vi "Framework PPL Test.vi"() -> ()   [LabVIEW 2017]
uses:
  Built/DSF.Engine.lvlibp/Shared/Typedefs/DSF.Shared.Typedefs.Data Type.ctl
  Built/DSF.Engine.lvlibp/Shared/Typedefs/DSF.Shared.Typedefs.Direction.ctl
  Built/DSF.Engine.lvlibp/Shared/Typedefs/DSF.Shared.Typedefs.Cycle Timing Factors.ctl
  Built/DSF.Engine.lvlibp/Engine/Classes/Framework/DSF.Engine.Framework.lvclass
  <vilib>/Platform/TimedLoop/XDataNode/timing_clust.ctl
  <vilib>/Platform/TimedLoop/XDataNode/nitl_modes.ctl
  <vilib>/Platform/TimedLoop/XDataNode/wakeup.ctl
  Built/DSF.Engine.lvlibp/Engine/Classes/Debug/DSF.Engine.Debug Flags.FIFO.lvclass
  Built/DSF.Engine.lvlibp/Engine/Classes/Debug/DSF.Engine.Debug Flags.lvclass
  Built/Memory Manager.lvlibp/1abvi3w/vi.lib/National Instruments/Memory Manager/Classes/Pointer/Memory.Pointer.New.4B.vi
  Built/Memory Manager.lvlibp/1abvi3w/vi.lib/National Instruments/Memory Manager/Classes/Pointer/Memory.Pointer.Write.0D.U32.vi
  Built/Memory Manager.lvlibp/1abvi3w/vi.lib/National Instruments/Memory Manager/Classes/Pointer/Memory.Pointer.New.1B.vi
  Built/Memory Manager.lvlibp/1abvi3w/vi.lib/National Instruments/Memory Manager/Classes/Pointer/Memory.Pointer.Write.0D.Bool.vi
  Built/Memory Manager.lvlibp/1abvi3w/vi.lib/National Instruments/Memory Manager/Classes/Pointer/Memory.Pointer.Read.0D.Bool.vi
  Built/Memory Manager.lvlibp/1abvi3w/vi.lib/National Instruments/Memory Manager/Classes/Pointer/Memory.Pointer.Read.0D.I32.vi
  Built/Memory Manager.lvlibp/1abvi3w/vi.lib/National Instruments/Memory Manager/Classes/Pointer/Memory.Pointer.Read.0D.U32.vi
  Built/Memory Manager.lvlibp/1abvi3w/vi.lib/National Instruments/Memory Manager/Classes/Pointer/Memory.Pointer.Write.0D.I32.vi
  <vilib>/platform/TimedLoop/XDataNode/XDataNode.xnode
  <vilib>/Platform/TimedLoop/XDataNode/XDNodeRunTimeDep.lvlib
  Built/Memory Manager.lvlibp/1abvi3w/vi.lib/National Instruments/Memory Manager/Classes/Pointer/Memory.Pointer.lvclass
  Built/DSF.Engine.lvlibp/Shared/Classes/Framework/DSF.Shared.Configuration.Framework.lvclass
  Built/DSF.Engine.lvlibp/Engine/Classes/Pointer/DSF.Engine.Pointer.DBL.lvclass
  Built/DSF.Engine.lvlibp/Engine/Classes/Status/DSF.Engine.Status.Framework.lvclass
  Built/DSF.Engine.lvlibp/Engine/Classes/Status/DSF.Engine.Status.Framework.Performance.lvclass
  Built/DSF.Engine.lvlibp
panel:
  out "UDP Rx Port 4":u16
  out "UDP Rx Bytes 4":i32
  out "UDP Rx Count 4":i32
  out "UDP Rx Port 3":u16
  out "UDP Rx Bytes 3":i32
  out "UDP Rx Count 3":i32
  in  "infinite timeouts":bool
  out "Framework Error":errorcluster
  out "Tx duration":u32 format="%d us"
  out "Rx duration":u32 format="%d us"
  out "Actual PCL Frequency":dbl format="%.0pHz"
  out "UDP Rx Count 2":i32
  out "UDP Rx Count 1":i32
  out "UDP Rx Port 2":u16
  out "UDP Rx Bytes 2":i32
  out "UDP Rx Bytes 1":i32
  out "UDP Rx Port 1":u16
  in  "Transceiver Count":i32=4
  in  "Plugins":T4(array[cluster])=[{"plugin class"="udp", "channel count per transfer"=100, "transfer configs per group"=[{"random types?"=FALSE, "non-random type"=enum."DBL"}], "group configs"=[{"direction"=enum."Tx", "timing"={"Priority"=100, "Decimation"=1, "Offset"=0}}, {"direction"=enum."Tx", "timing"={"Priority"=100, "Decimation"=2, "Offset"=0}}, {"direction"=enum."Tx", "timing"={"Priority"=100, "Decimation"=3, "Offset"=0}}, {"direction"=enum."Tx", "timing"={"Priority"=100, "Decimation"=4, "Offset"=0}}], "plugin timing"={"Priority"=100, "Decimation"=1, "Offset"=0}}]
  in  "Configuration Path":path=path "C:/Users/Admin/Desktop/test.json"
  out "Framework Iteration":i32 format="%d cycles"
  out "Actual Period":u32 format="%d us"
  in  "Target PCL Frequency":dbl=100.0 caption="Target Period" format="%.0pHz"
  in  "stop":bool
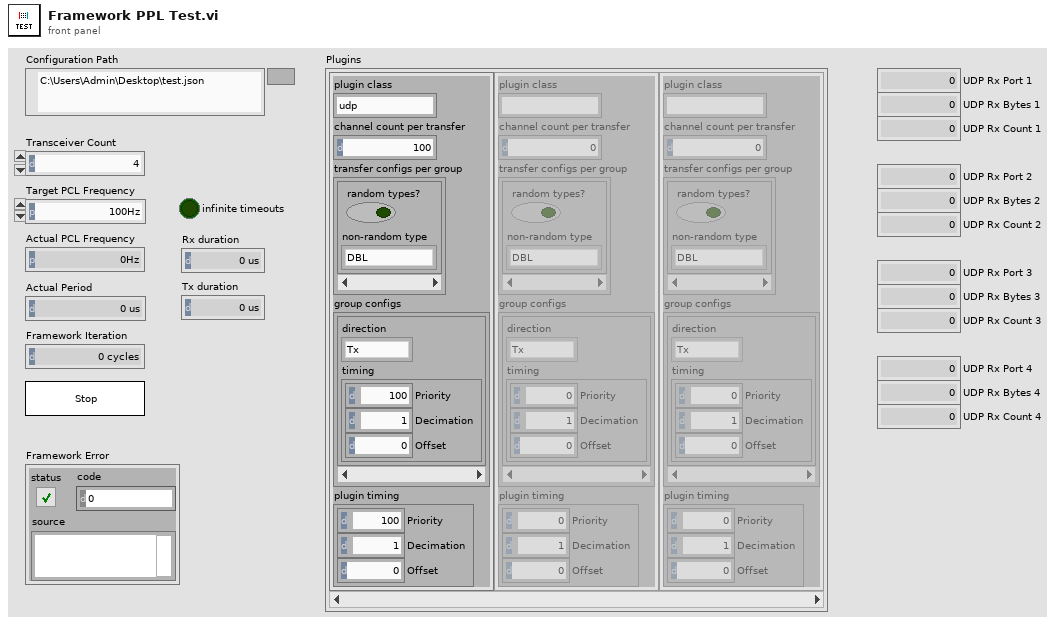
[diagram p1: front panel]
types:
  T1 = typedef "DSF.Engine.lvlibp/DSF.Shared.Typedefs.Data Type.ctl" = enum8{"Bool", "SGL", "DBL", "I8", "I16", "I32", "I64", "U8", "U16", "U32", "U64"}
  T2 = typedef "DSF.Engine.lvlibp/DSF.Shared.Typedefs.Direction.ctl" = enum8{"Tx", "Rx"}
  T3 = typedef "DSF.Engine.lvlibp/DSF.Shared.Typedefs.Cycle Timing Factors.ctl" = cluster{"Priority":u64, "Decimation":u64, "Offset":u64}
  T4 = cluster{"plugin class":string, "channel count per transfer":i32, "transfer configs per group":cluster{"random types?":bool, "non-random type":T1}[], "group configs":cluster{"direction":T2, "timing":T3}[], "plugin timing":T3}[]
  T5 = typedef "DSF.Engine.lvlibp/DSF.Shared.Refactor.Typedefs.Framework Configuration.Aggregate.ctl" = cluster{"Plugins":T6[]}
  T6 = typedef "DSF.Engine.lvlibp/DSF.Shared.Refactor.Typedefs.Plugin Configuration.Aggregate.ctl" = cluster{"name":string, "class":string, "cycle timing":T3, "Transfer Groups":T7[]}
  T7 = typedef "DSF.Engine.lvlibp/DSF.Shared.Refactor.Typedefs.Transfer Group Configuration.Aggregate.ctl" = cluster{"name":string, "direction":T2, "cycle timing":T3, "Transfers":T8[]}
  T8 = typedef "DSF.Engine.lvlibp/DSF.Shared.Refactor.Typedefs.Transfer Configuration.ctl" = cluster{"name":string, "byte order":T9, "channel configurations":T10[]}
  T9 = typedef "DSF.Engine.lvlibp/DSF.Shared.Typedefs.Byte Order.ctl" = enum8{"big-endian", "little-endian"}
  T10 = typedef "DSF.Engine.lvlibp/DSF.Shared.Refactor.Typedefs.Channel Array Configuration.ctl" = cluster{"name":string, "data type":T1, "count":u64, "buffer offset":u64, "engine offset":u64}
  T11 = typedef "XDNodeRunTimeDep.lvlib/timing_clust.ctl" = cluster{"Expected End [f-1]":u64, "Actual End [f-1]":u64, "Finished Late? [f-1]":bool, "Expected End [i-1]":u64, "Actual End [i-1]":u64, "Finished Late? [i-1]":bool, "Expected Start [i]":u64, "Actual Start [i]":u64, "Expected Start [f]":u64, "Actual Start [f]":u64, "Source Name":string, "Structure Name":string, "Period":i64, "Deadline":i64, "Offset":i64, "Start":i64, "Priority":i32, "Timeout":i32, "Mode":T12, "Wakeup Reason":T13, "Error":errorcluster, "Source Type":string, "Secondary Source Type":string, "Global End Time":u64, "Global Start Time":u64, "Frame Duration":u64, "Iteration Duration":u64, "Assigned CPU":i32, "I/O Scan Engine Mode":u32}
  T12 = typedef "XDNodeRunTimeDep.lvlib/nitl_modes.ctl" = enum32{"No Change", "Process missed periods, maintain original phase", "Discard missed periods, maintain original phase", "Process missed periods, ignore original phase", "Discard missed periods, ignore original phase"}
  T13 = typedef "XDNodeRunTimeDep.lvlib/wakeup.ctl" = enum32{"Normal", "Aborted", "Asynchronous wakeup", "Timing source error", "Timed loop error", "Timeout"}
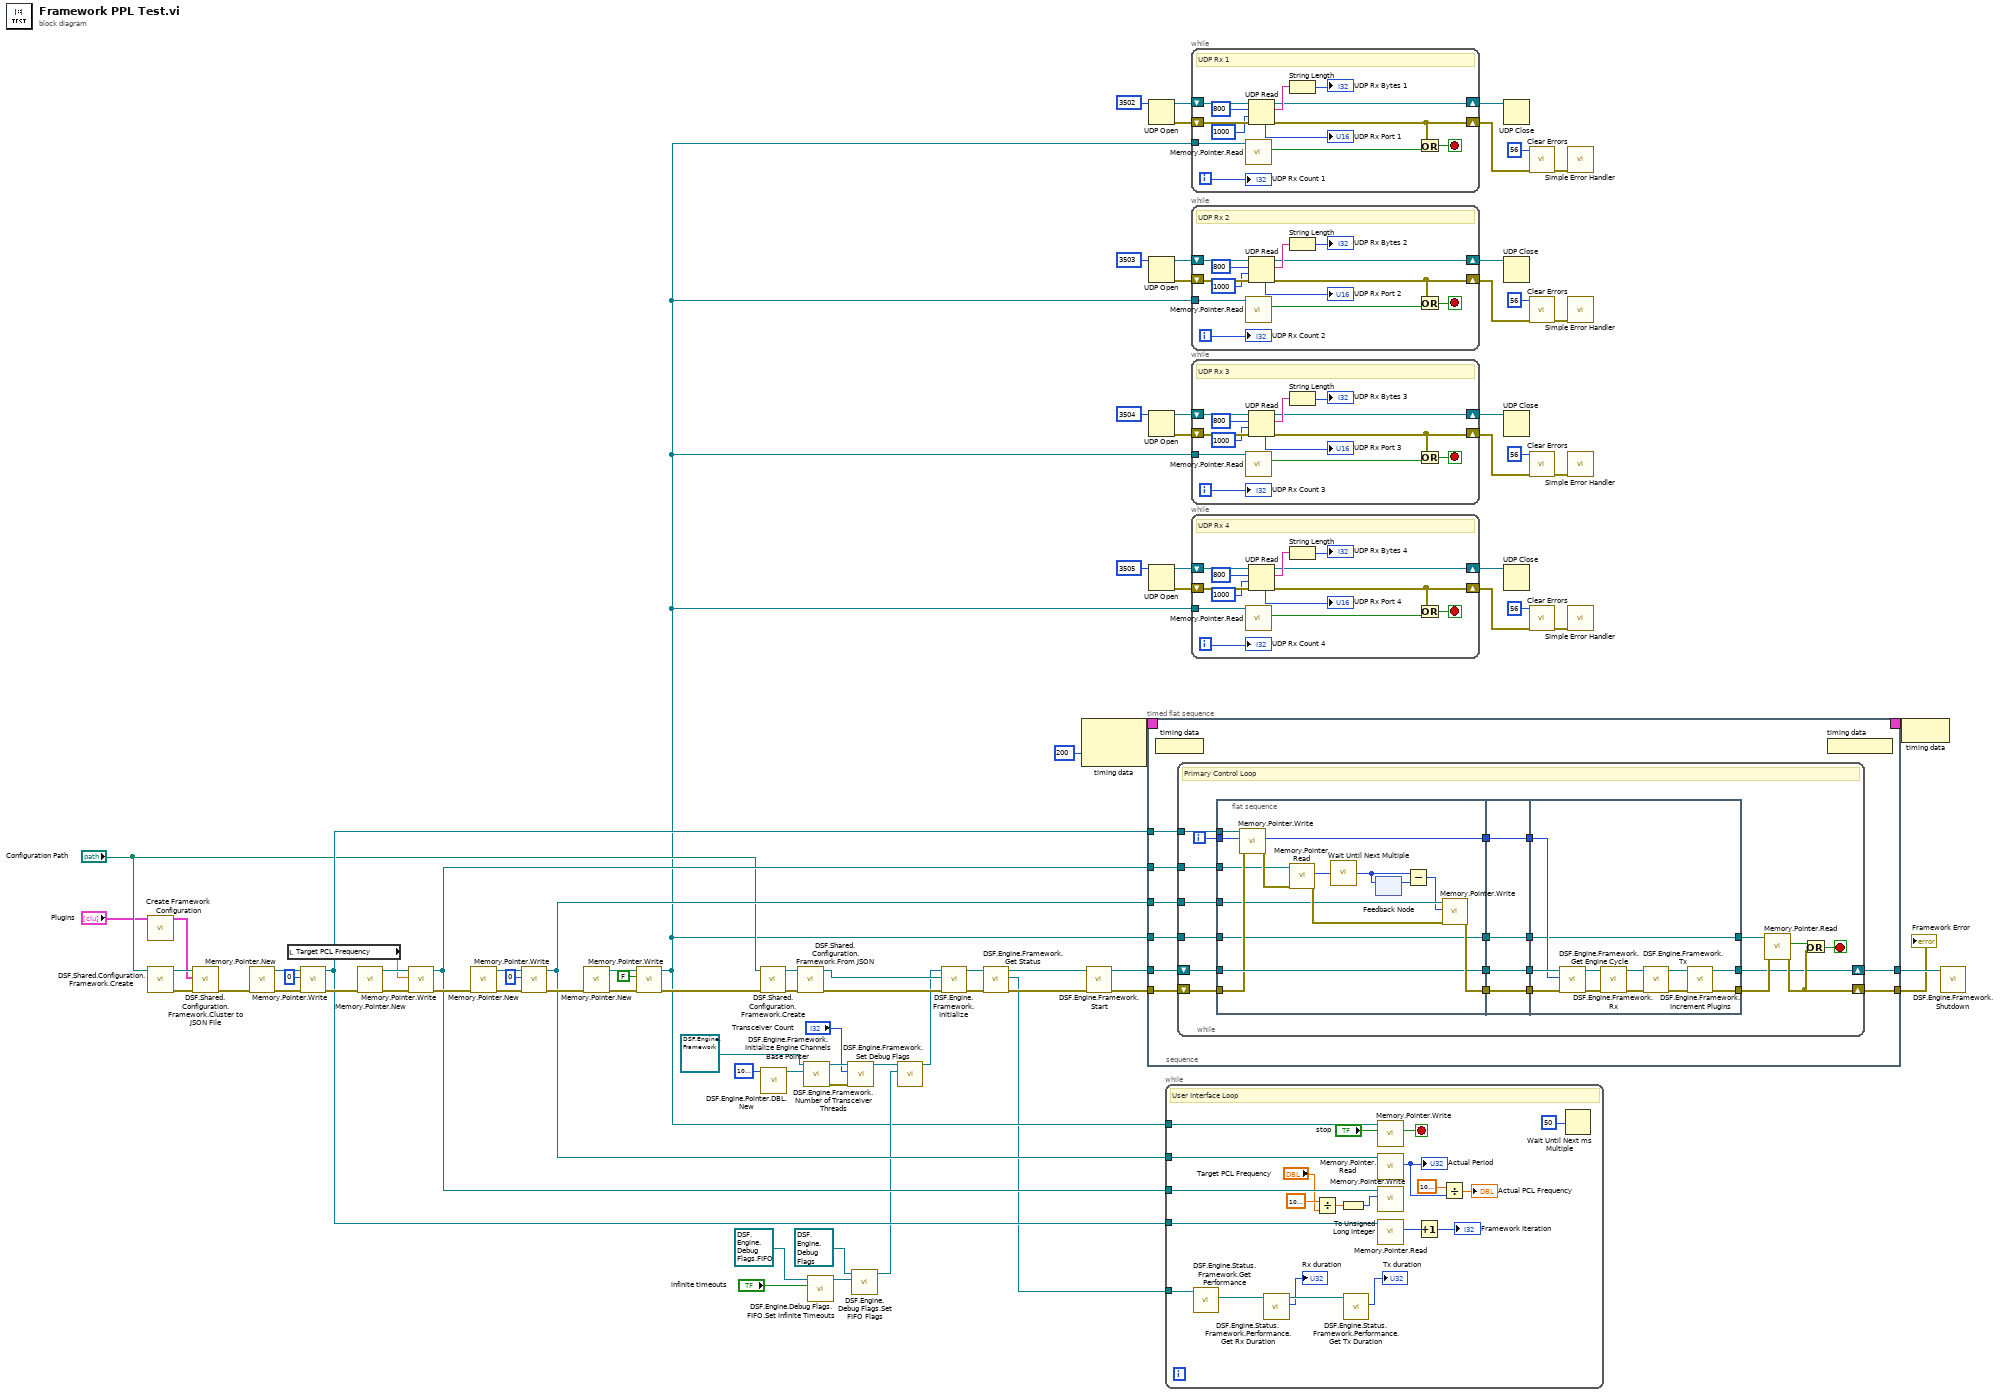
[diagram p0: block diagram]
diagram:
  n1 = call "Create Framework Configuration.vi"("Plugins"="Plugins") -> ("Framework Configuration"=w52:T5)  [unwired: 10 in]
  n2 = call "DSF.Shared.Configuration.Framework.Create.vi"("configuration path"="Configuration Path") -> ("error out"=w53:errorcluster, "Framework Configuration"=w54:refnum<class "DSF.Shared.Configuration.Framework.lvclass">)  [unwired: 9 in]
  n3 = call "DSF.Shared.Configuration.Framework.Cluster to JSON File.vi"("error in (no error)"=w53, "Framework Configuration"=w52, "Framework Configuration in"=w54) -> ("error out"=w51:errorcluster)  [unwired: 7 in, 1 out]
  n4 = call-poly "Memory.Pointer.New.vi"("error in (no error)"=w51) -> ("error out"=w60:errorcluster, "Pointer"=w62:refnum<class "Memory.Pointer.lvclass">)  [unwired: 9 in]
  n5 = local read "Target PCL Frequency"() -> (w70:dbl)
  n6 = call-poly "Memory.Pointer.Write.vi"("error in (no error)"=w60, "value"=u32 0, "Pointer in"=w62) -> ("error out"=w59:errorcluster, "Pointer out"=w56:refnum<class "Memory.Pointer.lvclass">)  [unwired: 5 in, 2 out]
  n7 = call-poly "Memory.Pointer.New.vi"("error in (no error)"=w59) -> ("error out"=w69:errorcluster, "Pointer"=w71:refnum<class "Memory.Pointer.lvclass">)  [unwired: 9 in]
  n8 = call-poly "Memory.Pointer.Write.vi"("error in (no error)"=w69, "value"=w70, "Pointer in"=w71) -> ("error out"=w68:errorcluster, "Pointer out"=w63:refnum<class "Memory.Pointer.lvclass">)  [unwired: 5 in, 2 out]
  n9 = call-poly "Memory.Pointer.New.vi"("error in (no error)"=w68) -> ("error out"=w66:errorcluster, "Pointer"=w72:refnum<class "Memory.Pointer.lvclass">)  [unwired: 9 in]
  n10 = call-poly "Memory.Pointer.Write.vi"("error in (no error)"=w66, "value"=u32 0, "Pointer in"=w72) -> ("error out"=w65:errorcluster, "Pointer out"=w64:refnum<class "Memory.Pointer.lvclass">)  [unwired: 5 in, 2 out]
  n11 = call-poly "Memory.Pointer.New.vi"("error in (no error)"=w65) -> ("error out"=w75:errorcluster, "Pointer"=w74:refnum<class "Memory.Pointer.lvclass">)  [unwired: 9 in]
  n12 = call-poly "Memory.Pointer.Write.vi"("error in (no error)"=w75, "value"=FALSE, "Pointer in"=w74) -> ("error out"=w55:errorcluster, "Pointer out"=w4:refnum<class "Memory.Pointer.lvclass">)  [unwired: 5 in, 2 out]
  n13 = call "DSF.Shared.Configuration.Framework.Create.vi"("error in (no error)"=w55, "configuration path"="Configuration Path") -> ("error out"=w57:errorcluster, "Framework Configuration"=w58:refnum<class "DSF.Shared.Configuration.Framework.lvclass">)  [unwired: 8 in]
  n14 = call "DSF.Engine.Pointer.DBL.New.vi"("channel count"=u64 1000000) -> ("DBL Pointer out"=w47:refnum<class "DSF.Engine.Pointer.DBL.lvclass">)  [unwired: 9 in, 1 out]
  n15 = call "DSF.Shared.Configuration.Framework.From JSON.vi"("error in (no error)"=w57, "Framework Configuration in"=w58) -> ("error out"=w82:errorcluster, "Framework Configuration out"=w48:refnum<class "DSF.Shared.Configuration.Framework.lvclass">)  [unwired: 8 in]
  n16 = call-dynamic "DSF.Engine.Framework.Initialize Engine Channels Base Pointer.vi"("Engine Channels Pointer"=w47, "Framework in"=refnum<class "DSF.Engine.Framework.lvclass"> refnum) -> ("error out"=w41:errorcluster, "Framework out"=w44:refnum<class "DSF.Engine.Framework.lvclass">)  [unwired: 8 in]
  n17 = call "DSF.Engine.Debug Flags.FIFO.Set Infinite Timeouts.vi"("infinite timeouts"="infinite timeouts", "FIFO Debug Flags in"=refnum<class "DSF.Engine.Debug Flags.FIFO.lvclass"> refnum) -> ("FIFO Debug Flags out"=w26:refnum<class "DSF.Engine.Debug Flags.FIFO.lvclass">)  [unwired: 9 in]
  n18 = call "DSF.Engine.Framework.Number of Transceiver Threads.vi"("error in (no error)"=w41, "transceiver count"="Transceiver Count", "Framework in"=w44) -> ("Framework out"=w28:refnum<class "DSF.Engine.Framework.lvclass">)  [unwired: 7 in, 1 out]
  n19 = call "DSF.Engine.Debug Flags.Set FIFO Flags.vi"("FIFO"=w26, "Debug Flags in"=refnum<class "DSF.Engine.Debug Flags.lvclass"> refnum) -> ("Debug Flags out"=w22:refnum<class "DSF.Engine.Debug Flags.lvclass">)  [unwired: 9 in]
  n20 = call "DSF.Engine.Framework.Set Debug Flags.vi"("Debug Flags"=w22, "Framework in"=w28) -> ("Framework out"=w27:refnum<class "DSF.Engine.Framework.lvclass">)  [unwired: 9 in]
  n21 = call "DSF.Engine.Framework.Initialize.vi"("error in (no error)"=w82, "Framework Configuration"=w48, "Framework type"=w27) -> ("error out"=w21:errorcluster, "Framework out"=w3:refnum<class "DSF.Engine.Framework.lvclass">)  [unwired: 7 in]
  n22 = call "DSF.Engine.Framework.Get Status.vi"("Framework in"=w3) -> ("Status"=w1:refnum<class "DSF.Engine.Status.Framework.lvclass">, "Framework out"=w2:refnum<class "DSF.Engine.Framework.lvclass">)  [unwired: 9 in]
  n23 = node-c288(200 ("Priority")) -> (w77:T11)  [unwired: 1 in]
  n24 = call "DSF.Engine.Framework.Start.vi"("error in (no error)"=w21, "Framework in"=w2) -> ("error out"=w80:errorcluster, "Framework out"=w81:refnum<class "DSF.Engine.Framework.lvclass">)  [unwired: 8 in]
  n25 = timed-sequence {
    timing: w77 -> [_]
    timing-out: [_] -> w76
    tunnel: w81 -> [w90]
    tunnel: w80 -> [w89]
    tunnel: [w88] -> w79
    tunnel: [w87] -> w78
    tunnel: w4 -> [w86]
    tunnel: w63 -> [w85]
    tunnel: w64 -> [w84]
    tunnel: w56 -> [w83]
    n26 = timed-flat-sequence {
      tunnel: w90 -> [w98]
      tunnel: w89 -> [w97]
      tunnel: [w96] -> w88
      tunnel: [w95] -> w87
      tunnel: w86 -> [w94]
      tunnel: w85 -> [w93]
      tunnel: w84 -> [w92]
      tunnel: w83 -> [w91]
      n27 = node-c288() -> ()  [unwired: 1 in]
      n28 = while {
        shift-right: [w109] -> w96
        shift-left: w98 -> [w118]
        shift-right: [w111] -> w95
        shift-left: w97 -> [w119]
        tunnel: w94 -> [w117]
        tunnel: w93 -> [w115]
        tunnel: w92 -> [w114]
        tunnel: w91 -> [w108]
        i -> [w107]
        stop <- w110 stop-if-true
        # "Primary Control Loop"
        n29 = flat-sequence {
          tunnel: w119 -> [w127]
          tunnel: w118 -> [w132]
          tunnel: w117 -> [w123]
          tunnel: [w133] -> w106
          tunnel: [w132] -> w104
          tunnel: [w123] -> w102
          tunnel: w115 -> [w125]
          tunnel: w114 -> [w124]
          tunnel: w108 -> [w129]
          tunnel: w107 -> [w128]
          tunnel: [w120] -> w100
          tunnel: w106 -> [w138]
          tunnel: [w138] -> w105
          tunnel: w104 -> [w137]
          tunnel: [w137] -> w103
          tunnel: w102 -> [w136]
          tunnel: [w136] -> w101
          tunnel: w100 -> [w135]
          tunnel: [w135] -> w99
          tunnel: w105 -> [w147]
          tunnel: w103 -> [w148]
          tunnel: w101 -> [w139]
          tunnel: w99 -> [w146]
          tunnel: [w139] -> w116
          tunnel: [w143] -> w109
          tunnel: [w142] -> w113
          frame #0 {
            n30 = call-poly "Memory.Pointer.Write.vi"("error in (no error)"=w127, "value"=w128, "Pointer in"=w129) -> ("error out"=w126:errorcluster, "value"=w120:i32)  [unwired: 5 in, 2 out]
            n31 = call-poly "Memory.Pointer.Read.vi"("error in (no error)"=w126, "Pointer in"=w125) -> ("error out"=w130:errorcluster, "value out"=w131:u32)  [unwired: 6 in, 2 out]
            n32 = call "Wait Until Next Multiple"("Count(uSec)"=w131) -> ("Tick Count(uSec)"=w121:u32)
            n33 = feedback #1() -> (w134:u32)  [unwired: 1 in]
            n34 = feedback-in #1(w121) -> ()
            n35 = Subtract(x=w121, y=w134) -> (x-y=w122:u32)
            n36 = call-poly "Memory.Pointer.Write.vi"("error in (no error)"=w130, "value"=w122, "Pointer in"=w124) -> ("error out"=w133:errorcluster)  [unwired: 5 in, 3 out]
          }
          frame #1 {
          }
          frame #2 {
            n37 = call "DSF.Engine.Framework.Get Engine Cycle.vi"("error in (no error)"=w147, "iteration"=w146, "Framework in"=w148) -> ("error out"=w140:errorcluster, "Framework out"=w141:refnum<class "DSF.Engine.Framework.lvclass">)  [unwired: 7 in]
            n38 = call "DSF.Engine.Framework.Rx.vi"("error in (no error)"=w140, "Framework in"=w141) -> ("error out"=w150:errorcluster, "Framework out"=w149:refnum<class "DSF.Engine.Framework.lvclass">)  [unwired: 8 in]
            n39 = call "DSF.Engine.Framework.Tx.vi"("error in (no error)"=w150, "Framework in"=w149) -> ("error out"=w144:errorcluster, "Framework out"=w145:refnum<class "DSF.Engine.Framework.lvclass">)  [unwired: 8 in]
            n40 = call "DSF.Engine.Framework.Increment Plugins.vi"("error in (no error)"=w144, "Framework in"=w145) -> ("error out"=w142:errorcluster, "Framework out"=w143:refnum<class "DSF.Engine.Framework.lvclass">)  [unwired: 8 in]
          }
        }
        n41 = call-poly "Memory.Pointer.Read.vi"("error in (no error)"=w113, "Pointer in"=w116) -> ("error out"=w111:errorcluster, "value out"=w112:bool)  [unwired: 6 in, 2 out]
        n42 = Or(x=w112, y=w111) -> (x .or. y?=w110:bool)
      }
      n43 = node-c288() -> ()  [unwired: 1 out]
    }
  }
  "Framework Error" <- w78
  n44 = UDP Open(11:u16 3502 ("port")) -> (port=w40:refnum<k16>, 0:w39:errorcluster)  [unwired: 4 in, 1 out]
  n45 = UDP Open(11:u16 3503 ("port")) -> (port=w35:refnum<k16>, 0:w36:errorcluster)  [unwired: 4 in, 1 out]
  n46 = UDP Open(11:u16 3504 ("port")) -> (port=w14:refnum<k16>, 0:w13:errorcluster)  [unwired: 4 in, 1 out]
  n47 = UDP Open(11:u16 3505 ("port")) -> (port=w7:refnum<k16>, 0:w6:errorcluster)  [unwired: 4 in, 1 out]
  n48 = while {
    tunnel: w4 -> [w172]
    tunnel: w64 -> [w167]
    tunnel: w63 -> [w168]
    tunnel: w56 -> [w159]
    tunnel: w1 -> [w157]
    stop <- w173 stop-if-true
    # "User Interface Loop"
    n49 = call "DSF.Engine.Status.Framework.Get Performance.vi"("Framework Status in"=w157) -> ("Framework Performance"=w156:refnum<class "DSF.Engine.Status.Framework.Performance.lvclass">)  [unwired: 9 in, 1 out]
    n50 = call "DSF.Engine.Status.Framework.Performance.Get Rx Duration.vi"("Framework Performance in"=w156) -> ("rx duration"=→"Rx duration":u32, "Framework Performance out"=w155:refnum<class "DSF.Engine.Status.Framework.Performance.lvclass">)  [unwired: 8 in, 1 out]
    n51 = Divide(x=1000000.0 ("y"), y="Target PCL Frequency") -> (x/y=w163:dbl)
    n52 = To Unsigned Long Integer(number=w163) -> (unsigned 32bit integer=w161:u32)
    n53 = call "DSF.Engine.Status.Framework.Performance.Get Tx Duration.vi"("Framework Performance in"=w155) -> ("tx duration"=→"Tx duration":u32)  [unwired: 8 in, 2 out]
    n54 = call-poly "Memory.Pointer.Write.vi"("value"="stop", "Pointer in"=w172) -> ("value"=w173:bool)  [unwired: 6 in, 3 out]
    n55 = call-poly "Memory.Pointer.Read.vi"("Pointer in"=w167) -> ("value out"=w164:u32)  [unwired: 7 in, 3 out]
    "Actual Period" <- w164
    n56 = call-poly "Memory.Pointer.Write.vi"("value"=w161, "Pointer in"=w168) -> ()  [unwired: 6 in, 4 out]
    n57 = call-poly "Memory.Pointer.Read.vi"("Pointer in"=w159) -> ("value out"=w169:i32)  [unwired: 7 in, 3 out]
    n58 = Increment(x=w169) -> (x+1=→"Framework Iteration":i32)
    n59 = Divide(x=1000000.0, y=w164) -> (x/y=→"Actual PCL Frequency":dbl)
    n60 = Wait Until Next ms Multiple(millisecond multiple=u32 50 ("milliseconds to wait")) -> ()  [unwired: 1 out]
  }
  n61 = while {
    shift-right: [w177] -> w31
    shift-left: w39 -> [w185]
    shift-right: [w182] -> w34
    shift-left: w40 -> [w186]
    tunnel: w4 -> [w180]
    i -> [w175]
    stop <- w178 stop-if-true
    # "UDP Rx 1"
    n62 = call-poly "Memory.Pointer.Read.vi"("Pointer in"=w180) -> ("value out"=w179:bool)  [unwired: 7 in, 3 out]
    n63 = UDP Read(connection ID=w186, max size (548)=800, timeout ms (25000)=1000, 8:w185) -> (data out=w184:string, error out=w177:errorcluster, 3:w182:refnum<k16>, 4:→"UDP Rx Port 1":u16)  [unwired: 1 out]
    n64 = String Length(string=w184) -> (length=→"UDP Rx Bytes 1":i32)
    n65 = Or(x=w177, y=w179) -> (x .or. y?=w178:bool)
    "UDP Rx Count 1" <- w175
  }
  n66 = while {
    shift-right: [w190] -> w29
    shift-left: w36 -> [w198]
    shift-right: [w195] -> w33
    shift-left: w35 -> [w199]
    tunnel: w4 -> [w193]
    i -> [w188]
    stop <- w191 stop-if-true
    # "UDP Rx 2"
    n67 = call-poly "Memory.Pointer.Read.vi"("Pointer in"=w193) -> ("value out"=w192:bool)  [unwired: 7 in, 3 out]
    n68 = UDP Read(connection ID=w199, max size (548)=800, timeout ms (25000)=1000, 8:w198) -> (data out=w197:string, error out=w190:errorcluster, 3:w195:refnum<k16>, 4:→"UDP Rx Port 2":u16)  [unwired: 1 out]
    n69 = String Length(string=w197) -> (length=→"UDP Rx Bytes 2":i32)
    n70 = Or(x=w190, y=w192) -> (x .or. y?=w191:bool)
    "UDP Rx Count 2" <- w188
  }
  n71 = while {
    shift-right: [w203] -> w17
    shift-left: w13 -> [w211]
    shift-right: [w208] -> w15
    shift-left: w14 -> [w212]
    tunnel: w4 -> [w206]
    i -> [w201]
    stop <- w204 stop-if-true
    # "UDP Rx 3"
    n72 = call-poly "Memory.Pointer.Read.vi"("Pointer in"=w206) -> ("value out"=w205:bool)  [unwired: 7 in, 3 out]
    n73 = UDP Read(connection ID=w212, max size (548)=800, timeout ms (25000)=1000, 8:w211) -> (data out=w210:string, error out=w203:errorcluster, 3:w208:refnum<k16>, 4:→"UDP Rx Port 3":u16)  [unwired: 1 out]
    n74 = String Length(string=w210) -> (length=→"UDP Rx Bytes 3":i32)
    n75 = Or(x=w203, y=w205) -> (x .or. y?=w204:bool)
    "UDP Rx Count 3" <- w201
  }
  n76 = while {
    shift-right: [w216] -> w10
    shift-left: w6 -> [w224]
    shift-right: [w221] -> w8
    shift-left: w7 -> [w225]
    tunnel: w4 -> [w219]
    i -> [w214]
    stop <- w217 stop-if-true
    # "UDP Rx 4"
    n77 = call-poly "Memory.Pointer.Read.vi"("Pointer in"=w219) -> ("value out"=w218:bool)  [unwired: 7 in, 3 out]
    n78 = UDP Read(connection ID=w225, max size (548)=800, timeout ms (25000)=1000, 8:w224) -> (data out=w223:string, error out=w216:errorcluster, 3:w221:refnum<k16>, 4:→"UDP Rx Port 4":u16)  [unwired: 1 out]
    n79 = String Length(string=w223) -> (length=→"UDP Rx Bytes 4":i32)
    n80 = Or(x=w216, y=w218) -> (x .or. y?=w217:bool)
    "UDP Rx Count 4" <- w214
  }
  n81 = UDP Close(connection ID=w34) -> ()  [unwired: 1 in, 2 out]
  n82 = UDP Close(connection ID=w33) -> ()  [unwired: 1 in, 2 out]
  n83 = UDP Close(connection ID=w15) -> ()  [unwired: 1 in, 2 out]
  n84 = UDP Close(connection ID=w8) -> ()  [unwired: 1 in, 2 out]
  n85 = call <vilib>:"Clear Errors.vi"("error in (no error)"=w31, "specific error code to clear (0: all)"=56) -> ("error out"=w19:errorcluster)  [unwired: 4 in, 1 out]
  n86 = call <vilib>:"Clear Errors.vi"("error in (no error)"=w29, "specific error code to clear (0: all)"=56) -> ("error out"=w20:errorcluster)  [unwired: 4 in, 1 out]
  n87 = call <vilib>:"Clear Errors.vi"("error in (no error)"=w17, "specific error code to clear (0: all)"=56) -> ("error out"=w18:errorcluster)  [unwired: 4 in, 1 out]
  n88 = call <vilib>:"Clear Errors.vi"("error in (no error)"=w10, "specific error code to clear (0: all)"=56) -> ("error out"=w11:errorcluster)  [unwired: 4 in, 1 out]
  n89 = call <vilib>:"Simple Error Handler.vi"("error in (no error)"=w19) -> ()  [unwired: 4 in, 5 out]
  n90 = call <vilib>:"Simple Error Handler.vi"("error in (no error)"=w20) -> ()  [unwired: 4 in, 5 out]
  n91 = call <vilib>:"Simple Error Handler.vi"("error in (no error)"=w18) -> ()  [unwired: 4 in, 5 out]
  n92 = call <vilib>:"Simple Error Handler.vi"("error in (no error)"=w11) -> ()  [unwired: 4 in, 5 out]
  n93 = node-c288(w76) -> ()
  n94 = call "DSF.Engine.Framework.Shutdown.vi"("Framework in"=w79) -> ()  [unwired: 9 in, 2 out]
